vi "Untitled 17 (SubVI).vi"(10 "DENOMIDADOR  PADE":dbl[](array[numeric]), 11 "NUMERADOR  PADE":dbl[](array[numeric])) -> (1 "C":dbl[](array[numeric]), 2 "B":dbl[](array[numeric]), 3 "A":T1)   [LabVIEW 2020]
uses:
  <vilib>/Analysis/Matrix/Datatypes/RealMatrix.ctl
  <vilib>/Analysis/Matrix/Numeric/Conversions/Array To Matrix - RA.vi
  <vilib>/Analysis/7linalg.llb/Create Special Real Matrix.vi
  <vilib>/Analysis/Matrix/Numeric/Conversions/Array To Matrix - RA2.vi
  <vilib>/Analysis/Matrix/NI_Matrix.lvlib
  <vilib>/Analysis/NI_AALPro.lvlib
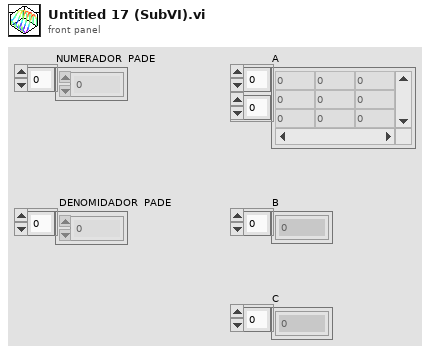
[diagram p1: front panel]
types:
  T1 = typedef "NI_Matrix.lvlib/RealMatrix.ctl" = dbl[][]
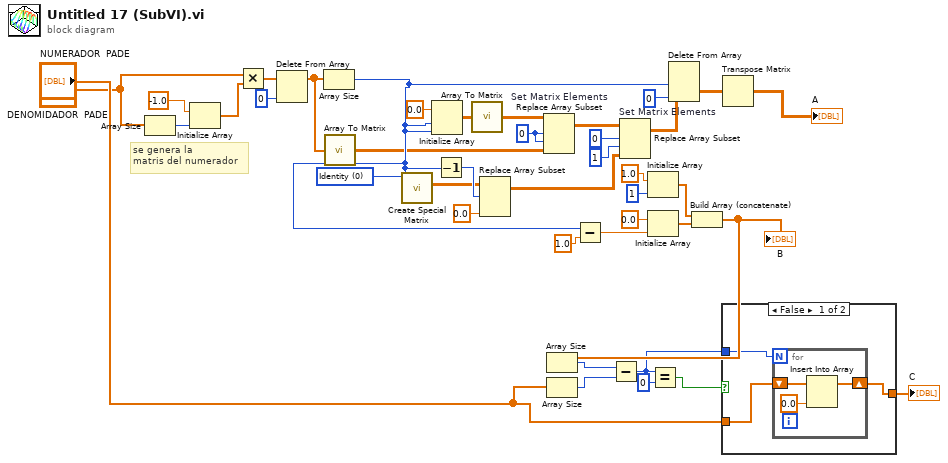
[diagram p0: block diagram]
diagram:
  w11 = 0 items=["Identity", "Diagonal", "Toeplitz", "Vandermonde", "Companion", "Hankel", "Hadamard", "Wilkinson", "Hilbert", "Inverse Hilbert", "Rosser", "Pascal"] ("matrix type")
  w7 = 0 ("disabled index (row)")
  # "se genera la \nmatris del numerador"
  n1 = Array Size(array="DENOMIDADOR  PADE") -> (size(s)=w1:i32)
  n2 = Initialize Array(-1.0 ("element"), w1) -> (w3:dbl[])
  n3 = Multiply(x="DENOMIDADOR  PADE", y=w3) -> (x*y=w4:dbl[])
  n4 = Delete From Array "Delete From Array"(array=w4, index=0) -> (array with subset deleted=w12:dbl[])  [unwired: 1 in, 1 out]
  n5 = Array Size(array=w12) -> (size(s)=w32:i32)
  n6 = call-poly <vilib>:"Array To Matrix.vi"("Real 1D Array"=w12) -> ("Real Matrix (Column Vector)"=w10:T1)
  n7 = call-poly <vilib>:"Create Special Matrix.vi"("matrix type"=w11, "matrix size"=w32) -> ("Special Matrix"=w16:T1)  [unwired: 3 in, 1 out]
  n8 = Initialize Array(0.0 ("element"), w32, w32) -> (w8:dbl[][])
  n9 = Decrement(x=w32) -> (x-1=w17:i32)
  n10 = call-poly <vilib>:"Array To Matrix.vi"("Real 2D Array"=w8) -> ("Real Matrix"=w9:T1)
  n11 = Replace Array Subset(array=w16, new element=0.0 ("new element/submatrix"), index (row)=w17) -> (w19:T1)  [unwired: 1 in]
  n12 = Replace Array Subset "Set Matrix Elements"(array=w9, new element=w10, index (row)=w7, index (col)=w7) -> (w15:T1)
  n13 = Array Size(array="NUMERADOR  PADE") -> (size(s)=w34:i32)
  n14 = Subtract(x=w32, y=1.0) -> (x-y=w30:dbl)
  n15 = Replace Array Subset "Set Matrix Elements"(array=w15, new element=w19, index (row)=0 ("disabled index (row)"), index (col)=1 ("disabled index (col)")) -> (w20:T1)
  n16 = Initialize Array(1.0 ("element"), 1 ("dimension size")) -> (w25:dbl[])
  n17 = Initialize Array(0.0 ("element"), w30) -> (w26:dbl[])
  n18 = Delete From Array(array=w20, length=w32, index (col)=0 ("disabled index (col)")) -> (deleted portion=w28:T1)  [unwired: 1 in, 1 out]
  n19 = Build Array (concatenate) "Build Array"(w25, w26) -> (w39:dbl[])
  "B" <- w39
  n20 = Array Size(array=w39) -> (size(s)=w33:i32)
  n21 = Subtract(x=w33, y=w34) -> (x-y=w37:i32)
  n22 = Equal?(x=w37, y=0) -> (x = y?=w36:bool)
  n23 = case shown="False" w36 {
    tunnel: "NUMERADOR  PADE" -> [w43 w47]
    tunnel: [w42 w47] -> w38
    tunnel: w37 -> [w41 _]
    frame False {
      n24 = for {
        N: w41 -> [_]
        shift-right: [w44] -> w42
        shift-left: w43 -> [w46]
        n25 = Insert Into Array(array=w46, new element=0.0 ("new element/subarray")) -> (w44:dbl[])  [unwired: 1 in]
      }
    }
    frame True {
    }
  }
  "C" <- w38
  n26 = Transpose Matrix(1:w28) -> (0:→"A":T1)
